vi "SuperNS_New.vi"(0 "reference in":refnum<class "SuperNS.lvclass">, 1 "Object name":string, 5 "error in":errorcluster, 6 "CreateMethod(Create or look up existing)":T4(ring)) -> (14 "reference out":refnum<class "SuperNS.lvclass">, 15 "NewObjectCreated":bool, 16 "DVRRefOut":refnum<data-value>, 19 "error out":errorcluster)   [LabVIEW 2020, in "SuperNS.lvclass"]
doc: "Copyright © 2008 - 2024 VI Technologies B.V. \nALL RIGHTS RESERVED"
uses:
  SuperNS.lvclass
  protected/ObjectAttributes.ctl
  <vilib>/dex/Stream Element Allocation Mode.ctl
  <vilib>/dex/Flush And Wait Empty Condition.ctl
  StreamDataType.ctl
  SuperNS.lvclass/SuperNS.ctl
panel:
  in  "DVRRef(Hidden)":refnum<data-value>
  in  "Data":T1 {"Flush Wait Condition" items=["All Elements Read From Stream", "All Elements Available for Reading"]; "Element Allocation Mode" items=["allocate as needed", "pre-allocate"]}
  in  "New":bool
  # "Copyright (c) 2024, VI Technologies B.V.\nAll rights reserved.\n\nRedistribution and use in source and binary forms, with or without modification, are permitted provided that \nthe following conditions are met:\n\n * Redistributions of source code must retain the above copyright notice, this list of conditions and the \nfollowing disclaimer.\n * Redistributions in binary form must reproduce the above copyright notice, this list of conditions and the \nfollowing disclaimer in the documentation and/or other materials provided with the distribution.\n * Neither the name of VI Technologies B.V. nor the names of its contributors may be used to endorse or \npromote products derived from this software without specific prior written permission.\n\nTHIS SOFTWARE IS PROVIDED BY THE COPYRIGHT HOLDERS AND CONTRIBUTORS \"AS IS\" AND ANY EXPRESS OR \nIMPLIED WARRANTIES, INCLUDING, BUT NOT LIMITED TO, THE IMPLIED WARRANTIES OF MERCHANTABILITY \nAND FITNESS FOR A PARTICULAR PURPOSE ARE DISCLAIMED. IN NO EVENT SHALL THE COPYRIGHT OWNER OR \nCONTRIBUTORS BE LIABLE FOR ANY DIRECT, INDIRECT, INCIDENTAL, SPECIAL, EXEMPLARY, OR CONSEQUENTIAL \nDAMAGES (INCLUDING, BUT NOT LIMITED TO, PROCUREMENT OF SUBSTITUTE GOODS OR SERVICES; LOSS OF \nUSE, DATA, OR PROFITS; OR BUSINESS INTERRUPTION) HOWEVER CAUSED AND ON ANY THEORY OF LIABILITY, \nWHETHER IN CONTRACT, STRICT LIABILITY, OR TORT (INCLUDING NEGLIGENCE OR OTHERWISE) ARISING IN ANY \nWAY OUT OF THE USE OF THIS SOFTWARE, EVEN IF ADVISED OF THE POSSIBILITY OF SUCH DAMAGE.\n\nFor more information, please visit https://www.vi-tech.nl or contact us at info@vi-tech.nl"
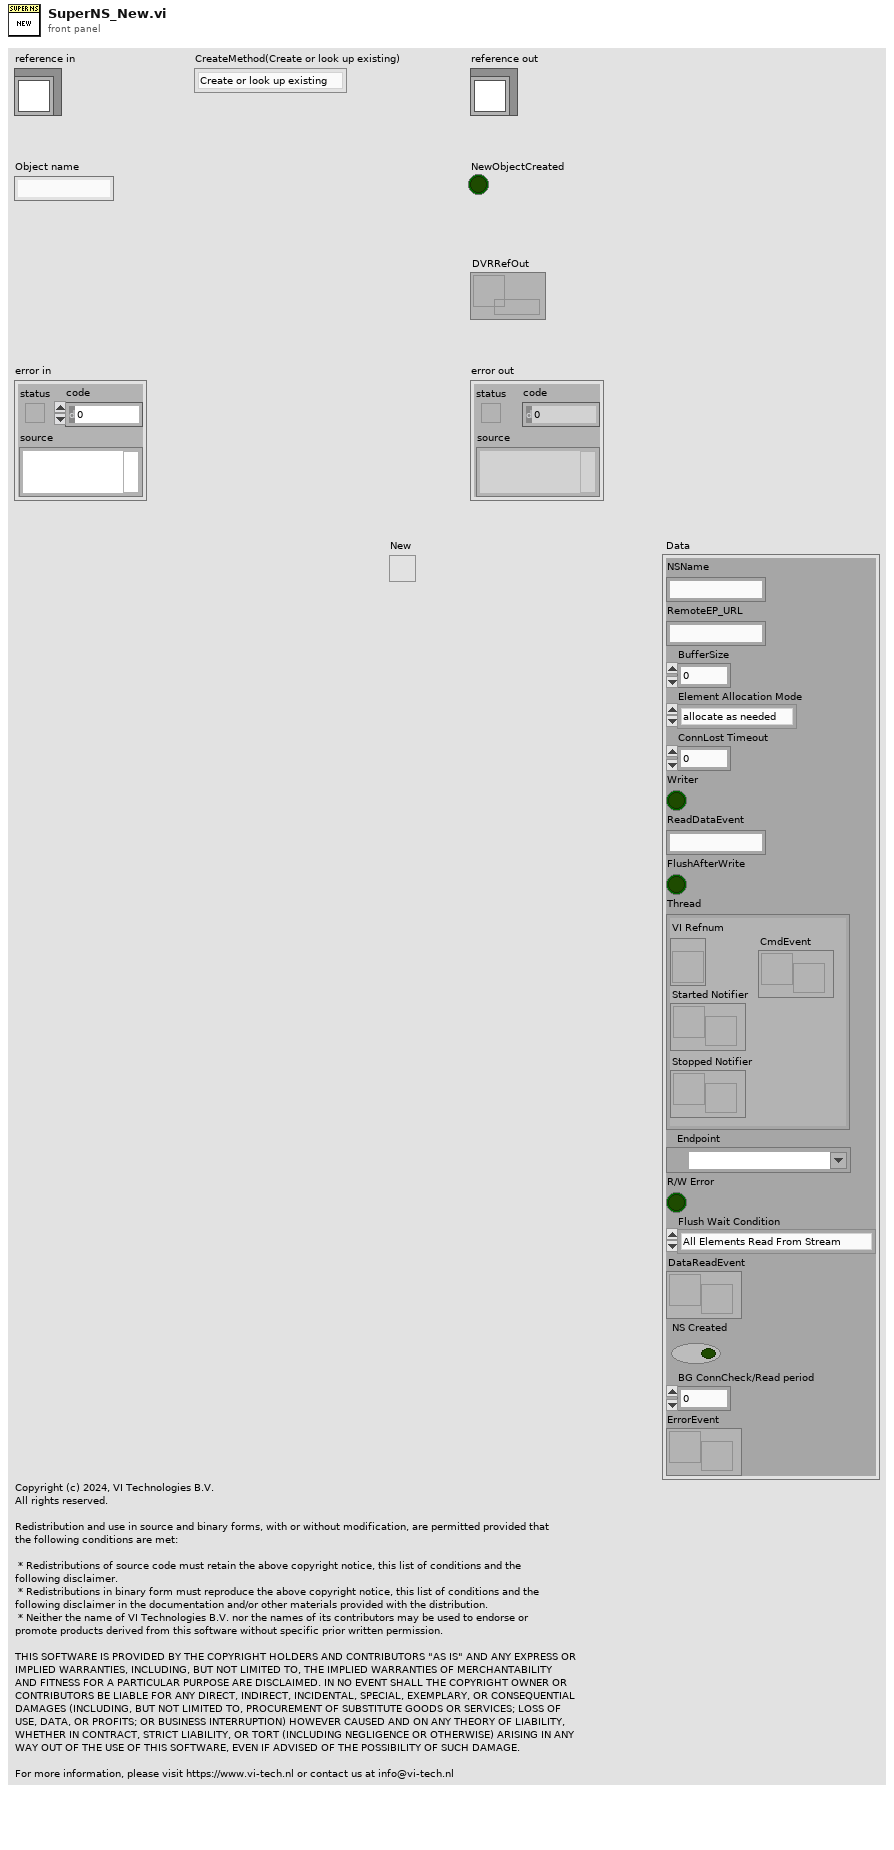
[diagram p1: front panel]
types:
  T1 = typedef "SuperNS.lvclass/ObjectAttributes.ctl" = cluster{"NSName":string, "RemoteEP_URL":string, "BufferSize":i32, "Element Allocation Mode":T2, "ConnLost Timeout":i32, "Writer":bool, "ReadDataEvent":string, "FlushAfterWrite":bool, "Thread":cluster{"VI Refnum":refnum<vi>, "Started Notifier":refnum<notifier>, "Stopped Notifier":refnum<notifier>, "CmdEvent":refnum<user-event>}, "Endpoint":refnum<k21>, "R/W Error":bool, "Flush Wait Condition":T3, "DataReadEvent":refnum<user-event>, "NS Created":bool, "BG ConnCheck/Read period":i32, "ErrorEvent":refnum<user-event>}
  T2 = typedef "Stream Element Allocation Mode.ctl" = u32
  T3 = typedef "Flush And Wait Empty Condition.ctl" = u8
  T4 = enum16{"Create or look up existing", "Look up existing"}
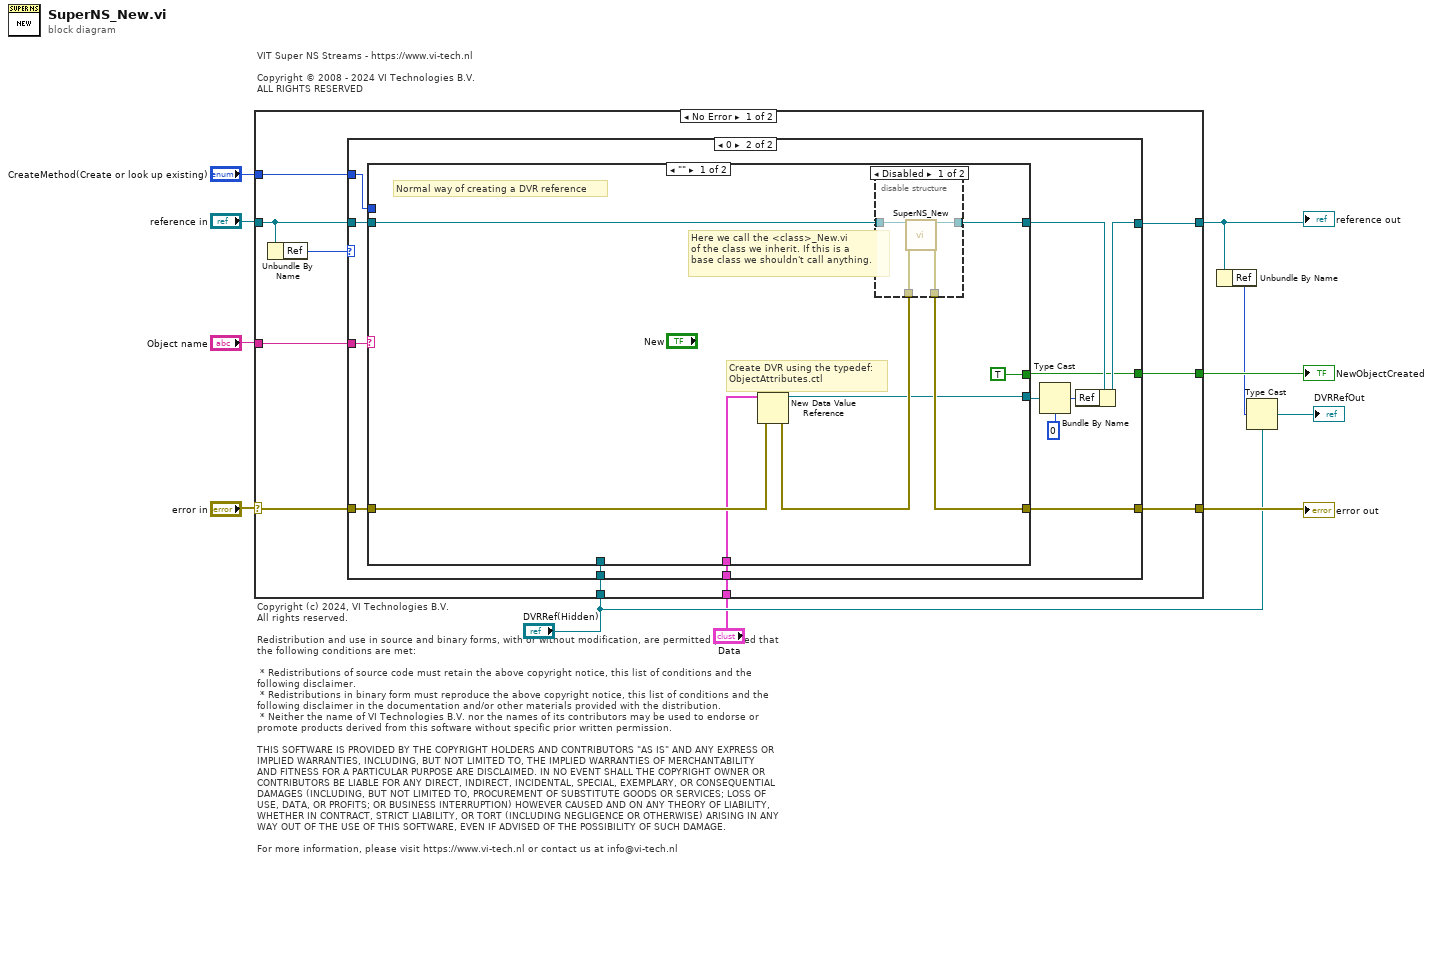
[diagram p0: block diagram]
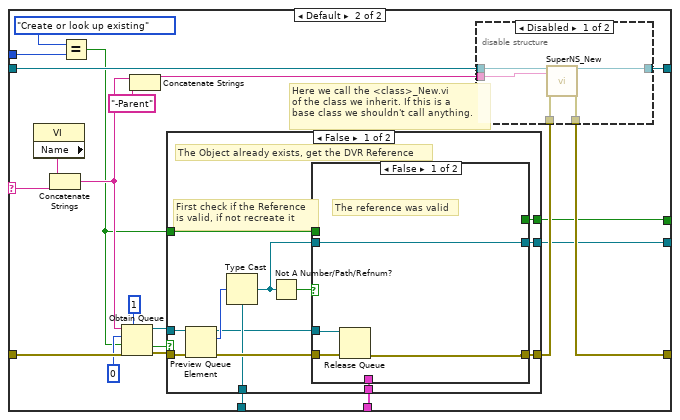
[diagram p4: hidden frame]
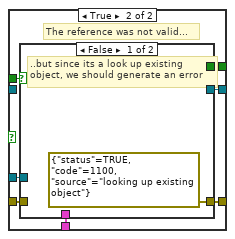
[diagram p5: hidden frame]
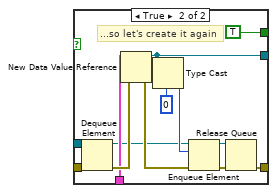
[diagram p6: hidden frame]
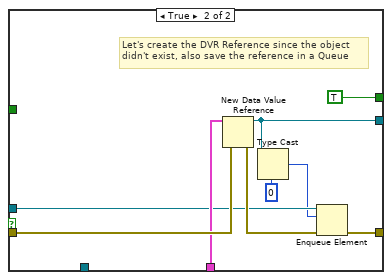
[diagram p7: hidden frame]
diagram:
  # "VIT Super NS Streams - https://www.vi-tech.nl\n\nCopyright © 2008 - 2024 VI Technologies B.V. \nALL RIGHTS RESERVED"
  # "Copyright (c) 2024, VI Technologies B.V.\nAll rights reserved.\n\nRedistribution and use in source and binary forms, with or without modification, are permitted provided that \nthe following conditions are met:\n\n * Redistributions of source code must retain the above copyright notice, this list of conditions and the \nfollowing disclaimer.\n * Redistributions in binary form must reproduce the above copyright notice, this list of conditions and the \nfollowing disclaimer in the documentation and/or other materials provided with the distribution.\n * Neither the name of VI Technologies B.V. nor the names of its contributors may be used to endorse or \npromote products derived from this software without specific prior written permission.\n\nTHIS SOFTWARE IS PROVIDED BY THE COPYRIGHT HOLDERS AND CONTRIBUTORS \"AS IS\" AND ANY EXPRESS OR \nIMPLIED WARRANTIES, INCLUDING, BUT NOT LIMITED TO, THE IMPLIED WARRANTIES OF MERCHANTABILITY \nAND FITNESS FOR A PARTICULAR PURPOSE ARE DISCLAIMED. IN NO EVENT SHALL THE COPYRIGHT OWNER OR \nCONTRIBUTORS BE LIABLE FOR ANY DIRECT, INDIRECT, INCIDENTAL, SPECIAL, EXEMPLARY, OR CONSEQUENTIAL \nDAMAGES (INCLUDING, BUT NOT LIMITED TO, PROCUREMENT OF SUBSTITUTE GOODS OR SERVICES; LOSS OF \nUSE, DATA, OR PROFITS; OR BUSINESS INTERRUPTION) HOWEVER CAUSED AND ON ANY THEORY OF LIABILITY, \nWHETHER IN CONTRACT, STRICT LIABILITY, OR TORT (INCLUDING NEGLIGENCE OR OTHERWISE) ARISING IN ANY \nWAY OUT OF THE USE OF THIS SOFTWARE, EVEN IF ADVISED OF THE POSSIBILITY OF SUCH DAMAGE.\n\nFor more information, please visit https://www.vi-tech.nl or contact us at info@vi-tech.nl"
  n1 = case shown="No Error" "error in" {
    selector: "error in" -> [w21 w128]
    tunnel: [w20 w128] -> w10
    tunnel: "CreateMethod(Create or look up existing)" -> [w18 _]
    tunnel: "Object name" -> [w19 _]
    tunnel: "Data" -> [w17 _]
    tunnel: "DVRRef(Hidden)" -> [w16 _]
    tunnel: "reference in" -> [w15 w127]
    tunnel: [w14 w127] -> w4
    tunnel: [w13 _] -> w6
    frame No Error {
      n2 = Unbundle By Name(w15) -> ("Ref"=w12:u32)
      n3 = case shown="0" w12 {
        tunnel: w21 -> [w23 w35]
        tunnel: w19 -> [_ w34]
        tunnel: w18 -> [_ w33]
        tunnel: [w23 w36] -> w20
        tunnel: w17 -> [_ w32]
        tunnel: w15 -> [w22 w30]
        tunnel: [w22 w31] -> w14
        tunnel: w16 -> [_ w28]
        tunnel: [_ w27] -> w13
        frame Default {
          # "The DVR reference has already been created, from this child class's <Child>_New.vi"
        }
        frame 0 {
          n4 = case shown="\"\"" w34 {
            selector: w34 -> [_ w60]
            tunnel: [w42 w71] -> w36
            tunnel: w33 -> [_ w67]
            tunnel: w32 -> [w41 w54]
            tunnel: [w40 w53] -> w25
            tunnel: w30 -> [w39 w66]
            tunnel: [w38 w65] -> w29
            tunnel: w28 -> [_ w55]
            tunnel: [TRUE ("created new?") w52] -> w27
            tunnel: w35 -> [w44 w72]
            frame "" {
              # "Create DVR using the typedef:\nObjectAttributes.ctl"
              # "Here we call the <class>_New.vi\nof the class we inherit. If this is a\nbase class we shouldn't call anything."
              # "Normal way of creating a DVR reference"
              n5 = New Data Value Reference(data value=w41, error in=w44) -> (data value reference=w40:refnum<data-value>, error out=w43:errorcluster)
              n6 = disable-structure shown="Disabled" {
                disable-tunnel: w39 -> [w46 w49]
                disable-tunnel: [w45 w49] -> w38
                disable-tunnel: w43 -> [w48 w50]
                disable-tunnel: [w47 w50] -> w42
                frame Disabled {
                  n7 = call "SuperNS_New.vi"("reference in"=w46, "error in"=w48) -> ("reference out"=w45:refnum<class "SuperNS.lvclass">, "error out"=w47:errorcluster)  [unwired: 14 in, 2 out]
                }
                frame Enabled {
                }
              }
            }
            frame Default {
              # "Here we call the <class>_New.vi\nof the class we inherit. If this is a\nbase class we shouldn't call anything."
              n8 = property class="VI"() -> ("Name"=w61:string)  [unwired: 2 in, 2 out]
              n9 = Concatenate Strings(w61, w60) -> (w59:string)
              n10 = Equal?(x=T4."Create or look up existing", y=w67) -> (x = y?=w56:bool)
              n11 = Obtain Queue(max queue size (-1, unlimited)=1, name (unnamed)=w59, element data type=u32 0 ("DataRef"), create if not found? (T)=w56, error in (no error)=w72) -> (queue out=w57:refnum<queue>, created new?=w58:bool, error out=w70:errorcluster)
              n12 = Concatenate Strings(w59, "-Parent" ("string")) -> (w62:string)
              n13 = case shown="False" w58 {
                tunnel: w70 -> [w85 w119]
                tunnel: w54 -> [w75 w116]
                tunnel: w57 -> [w82 w115]
                tunnel: [w83 w117] -> w69
                tunnel: [w77 w113] -> w53
                tunnel: w55 -> [w80 _]
                tunnel: [w74 TRUE] -> w52
                tunnel: w56 -> [w73 _]
                frame False {
                  # "First check if the Reference\nis valid, if not recreate it"
                  # "The Object already exists, get the DVR Reference"
                  n14 = Preview Queue Element(queue=w82, error in (no error)=w85) -> (queue out=w76:refnum<queue>, element=w81:u32, error out=w84:errorcluster)  [unwired: 1 in, 1 out]
                  n15 = Type Cast(type=w80, x=w81) -> (*(type *) &x=w78:refnum<data-value>)
                  n16 = Not A Number/Path/Refnum?(number/path/refnum=w78) -> (NaN/Path/Refnum?=w79:bool)
                  n17 = case shown="False" w79 {
                    tunnel: w84 -> [w89 w96]
                    tunnel: [w88 w95] -> w83
                    tunnel: w78 -> [w87 _]
                    tunnel: [w87 w92] -> w77
                    tunnel: w76 -> [w86 w94]
                    tunnel: w75 -> [_ w93]
                    tunnel: [_ w91] -> w74
                    tunnel: w73 -> [_ w90]
                    frame False {
                      # "The reference was valid"
                      n18 = Release Queue(queue=w86, error in (no error)=w89) -> (error out=w88:errorcluster)  [unwired: 1 in, 2 out]
                    }
                    frame True {
                      # "The reference was not valid..."
                      n19 = case shown="False" w90 {
                        tunnel: w94 -> [_ w105]
                        tunnel: w96 -> [_ w110]
                        tunnel: w93 -> [_ w102]
                        tunnel: [_ w100] -> w92
                        tunnel: [errorcluster {"status"=TRUE, "code"=1100, "source"="looking up existing object"} ("error out") w106] -> w95
                        tunnel: [_ TRUE] -> w91
                        frame False {
                          # "..but since its a look up existing\nobject, we should generate an error"
                        }
                        frame True {
                          # "...so let's create it again"
                          n20 = Dequeue Element(queue=w105, error in (no error)=w110) -> (queue out=w101:refnum<queue>, error out=w109:errorcluster)  [unwired: 1 in, 2 out]
                          n21 = New Data Value Reference(data value=w102, error in=w109) -> (data value reference=w100:refnum<data-value>, error out=w108:errorcluster)
                          n22 = Type Cast(type=u32 0 ("ObjectQueue"), x=w100) -> (*(type *) &x=w103:u32)
                          n23 = Enqueue Element(queue=w101, element=w103, error in (no error)=w108) -> (queue out=w98:refnum<queue>, error out=w107:errorcluster)  [unwired: 1 in, 1 out]
                          n24 = Release Queue(queue=w98, error in (no error)=w107) -> (error out=w106:errorcluster)  [unwired: 1 in, 2 out]
                        }
                      }
                    }
                  }
                }
                frame True {
                  # "Let's create the DVR Reference since the object\ndidn't exist, also save the reference in a Queue"
                  n25 = New Data Value Reference(data value=w116, error in=w119) -> (data value reference=w113:refnum<data-value>, error out=w118:errorcluster)
                  n26 = Type Cast(type=u32 0 ("ObjectQueue"), x=w113) -> (*(type *) &x=w112:u32)
                  n27 = Enqueue Element(queue=w115, element=w112, error in (no error)=w118) -> (error out=w117:errorcluster)  [unwired: 1 in, 2 out]
                }
              }
              n28 = disable-structure shown="Disabled" {
                disable-tunnel: w66 -> [w122 w125]
                disable-tunnel: [w121 w125] -> w65
                disable-tunnel: w62 -> [w120 _]
                disable-tunnel: w69 -> [w124 w126]
                disable-tunnel: [w123 w126] -> w71
                frame Disabled {
                  n29 = call "SuperNS_New.vi"("reference in"=w122, "Object name"=w120, "error in"=w124) -> ("reference out"=w121:refnum<class "SuperNS.lvclass">, "error out"=w123:errorcluster)  [unwired: 13 in, 2 out]
                }
                frame Enabled {
                }
              }
            }
          }
          n30 = Type Cast(type=u32 0 ("DataRef"), x=w25) -> (*(type *) &x=w24:u32)
          n31 = Bundle By Name(cluster=w29, "Ref"=w24) -> (w31:refnum<class "SuperNS.lvclass">)
        }
      }
    }
    frame Error {
    }
  }
  "error out" <- w10
  "reference out" <- w4
  "NewObjectCreated" <- w6
  n32 = Unbundle By Name(w4) -> ("Ref"=w5:u32)
  n33 = Type Cast(type="DVRRef(Hidden)", x=w5) -> (*(type *) &x=→"DVRRefOut":refnum<data-value>)
